vi "Builder.Main Thread.vi"(8 "error in (no error)":errorcluster, 10 "Thread Parameters":refnum<class "Thread Parameters.lvclass">, 11 "Builder in":refnum<class "Builder.lvclass">) -> (0 "error out":errorcluster, 3 "Builder out":refnum<class "Builder.lvclass">)   [LabVIEW 2016, in "DSF.Engine.lvlib" / "Builder.lvclass"]
uses:
  Builder.lvclass
  Thread Parameters/Thread Parameters.lvclass
  Thread Parameters/Thread Parameters.lvclass/Thread Parameters.ctl
  <vilib>/Platform/TimedLoop/XDataNode/timing_clust.ctl
  <vilib>/Platform/TimedLoop/XDataNode/nitl_modes.ctl
  <vilib>/Platform/TimedLoop/XDataNode/wakeup.ctl
  Builder.lvclass/Builder.ctl
  Interface/DSF.Engine.Interface.lvclass/DSF.Engine.Interface.ctl
  Interface/DSF.Engine.Interface.Builder.Response Data.ctl
  Interface/DSF.Engine.Interface.Builder.Response.ctl
  Interface/DSF.Engine.Interface.Builder.Read.Command.vi
  Interface/DSF.Engine.Interface.Builder.Write.Response.vi
  Interface/DSF.Engine.Interface.Get Command FIFO.vi
  Interface/DSF.Engine.Interface.RT FIFO.Read.vi
  Interface/DSF.Engine.Interface.RT FIFO.Write.vi
  Interface/DSF.Engine.Interface.Builder.lvclass
  C:/Git/Sourcetree/DSF/Source/Engine/Classes/Interface/DSF.Engine.Interface.lvclass
  <vilib>/platform/TimedLoop/XDataNode/XDataNode.xnode
  <vilib>/Platform/TimedLoop/XDataNode/XDNodeRunTimeDep.lvlib
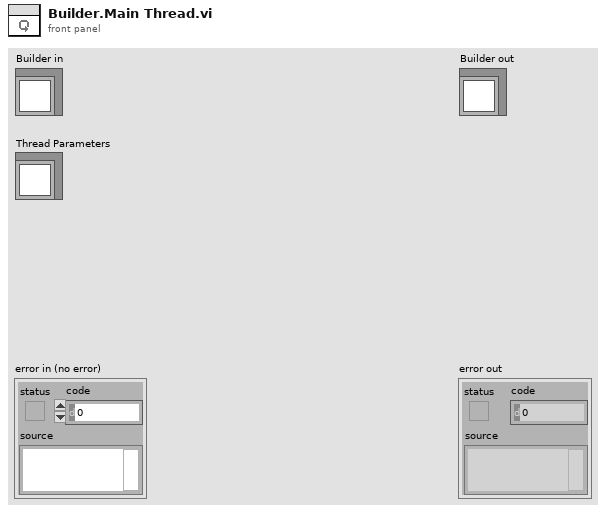
[diagram p1: front panel]
types:
  T1 = typedef "XDNodeRunTimeDep.lvlib/timing_clust.ctl" = cluster{"Expected End [f-1]":u64, "Actual End [f-1]":u64, "Finished Late? [f-1]":bool, "Expected End [i-1]":u64, "Actual End [i-1]":u64, "Finished Late? [i-1]":bool, "Expected Start [i]":u64, "Actual Start [i]":u64, "Expected Start [f]":u64, "Actual Start [f]":u64, "Source Name":string, "Structure Name":string, "Period":i64, "Deadline":i64, "Offset":i64, "Start":i64, "Priority":i32, "Timeout":i32, "Mode":T2, "Wakeup Reason":T3, "Error":errorcluster, "Source Type":string, "Secondary Source Type":string, "Global End Time":u64, "Global Start Time":u64, "Frame Duration":u64, "Iteration Duration":u64, "Assigned CPU":i32, "I/O Scan Engine Mode":u32}
  T2 = typedef "XDNodeRunTimeDep.lvlib/nitl_modes.ctl" = enum32{"No Change", "Process missed periods, maintain original phase", "Discard missed periods, maintain original phase", "Process missed periods, ignore original phase", "Discard missed periods, ignore original phase"}
  T3 = typedef "XDNodeRunTimeDep.lvlib/wakeup.ctl" = enum32{"Normal", "Aborted", "Asynchronous wakeup", "Timing source error", "Timed loop error", "Timeout"}
  T4 = typedef "DSF.Engine.lvlib/DSF.Engine.Interface.Builder.lvclass/DSF.Engine.Interface.Builder.Response Data.ctl" = cluster{"Response":T5, "Payload":u64}
  T5 = typedef "DSF.Engine.lvlib/DSF.Engine.Interface.Builder.lvclass/DSF.Engine.Interface.Builder.Response.ctl" = enum8{"General Ack", "Shutdown Ack"}
  T6 = typedef "DSF.Engine.lvlib/DSF.Engine.Interface.Builder.lvclass/DSF.Engine.Interface.Builder.Command Data.ctl" = cluster{"Command":T7, "Payload":u64}
  T7 = typedef "DSF.Engine.lvlib/DSF.Engine.Interface.Builder.lvclass/DSF.Engine.Interface.Builder.Command.ctl" = enum8{"Idle", "Initialize", "Build Buffer", "Parse Buffer", "Shutdown"}
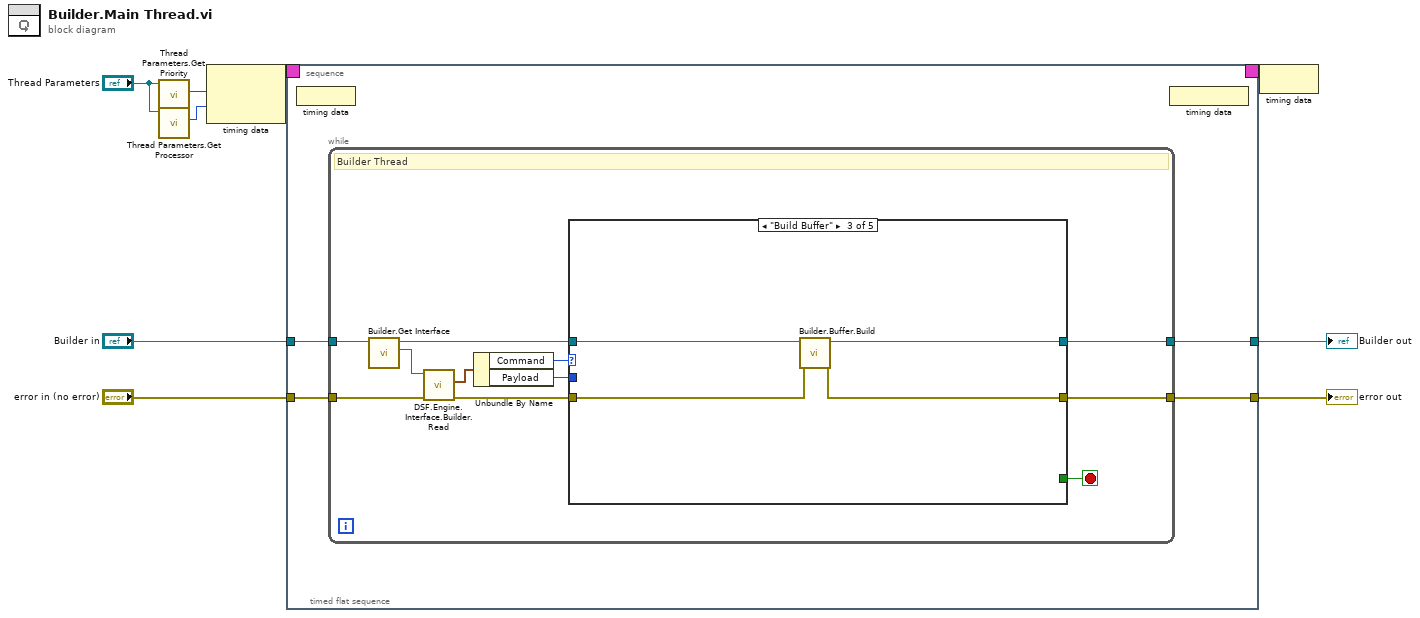
[diagram p0: block diagram]
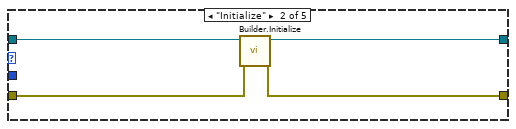
[diagram p3: hidden frame]
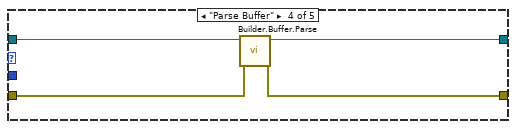
[diagram p4: hidden frame]
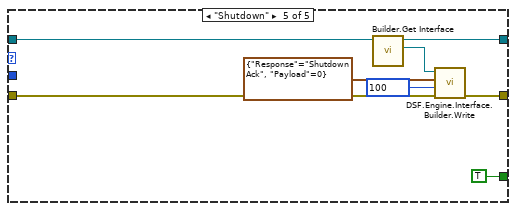
[diagram p5: hidden frame]
diagram:
  n1 = call "Thread Parameters.Get Priority.vi"("Thread Parameters in"="Thread Parameters") -> ("Priority"=w6:i32)  [unwired: 9 in, 1 out]
  n2 = call "Thread Parameters.Get Processor.vi"("Thread Parameters in"="Thread Parameters") -> ("Processor"=w5:i32)  [unwired: 9 in, 1 out]
  n3 = node-c288(w6, w5) -> (w8:T1)
  n4 = timed-sequence {
    timing: w8 -> [_]
    timing-out: [_] -> w7
    tunnel: "Builder in" -> [w12]
    tunnel: [w13] -> w4
    tunnel: "error in (no error)" -> [w11]
    tunnel: [w10] -> w2
    n5 = timed-flat-sequence {
      tunnel: [w17] -> w13
      tunnel: w12 -> [w15]
      tunnel: w11 -> [w16]
      tunnel: [w14] -> w10
      n6 = node-c288() -> ()  [unwired: 1 in]
      n7 = while {
        tunnel: w15 -> [w21]
        tunnel: [w25] -> w17
        tunnel: w16 -> [w29]
        tunnel: [w22] -> w14
        stop <- w20 stop-if-true
        # "Builder Thread"
        n8 = call "Builder.Get Interface.vi"("Builder in"=w21) -> ("Builder Interface"=w30:refnum<class "DSF.Engine.Interface.Builder.lvclass">, "Builder out"=w26:refnum<class "Builder.lvclass">)  [unwired: 9 in]
        n9 = call-poly "DSF.Engine.Interface.Builder.Read.vi"("error in (no error)"=w29, "Builder Interface in"=w30) -> ("error out"=w23:errorcluster, "command"=w28:T6)  [unwired: 5 in, 3 out]
        n10 = Unbundle By Name(w28) -> ("Command"=w27:T7, "Payload"=w24:u64)
        n11 = case shown="\"Build Buffer\"" w27 {
          tunnel: w26 -> [w32 w36 w40 w44 w52]
          tunnel: [w32 w35 w39 w43 w51] -> w25
          tunnel: w24 -> [_ _ _ _ _]
          tunnel: w23 -> [w31 w34 w38 w42 w47]
          tunnel: [w31 w33 w37 w41 w50] -> w22
          tunnel: [_ _ _ _ TRUE] -> w20
          frame "Idle", Default {
          }
          frame "Initialize" {
            n12 = call "Builder.Initialize.vi"("error in (no error)"=w34, "Builder in"=w36) -> ("error out"=w33:errorcluster, "Builder out"=w35:refnum<class "Builder.lvclass">)  [unwired: 8 in]
          }
          frame "Build Buffer" {
            n13 = call "Builder.Buffer.Build.vi"("error in (no error)"=w38, "Builder in"=w40) -> ("error out"=w37:errorcluster, "Builder out"=w39:refnum<class "Builder.lvclass">)  [unwired: 8 in]
          }
          frame "Parse Buffer" {
            n14 = call "Builder.Buffer.Parse.vi"("error in (no error)"=w42, "Builder in"=w44) -> ("error out"=w41:errorcluster, "Builder out"=w43:refnum<class "Builder.lvclass">)  [unwired: 8 in]
          }
          frame "Shutdown" {
            n15 = call "Builder.Get Interface.vi"("Builder in"=w52) -> ("Builder Interface"=w49:refnum<class "DSF.Engine.Interface.Builder.lvclass">, "Builder out"=w51:refnum<class "Builder.lvclass">)  [unwired: 9 in]
            n16 = call-poly "DSF.Engine.Interface.Builder.Write.vi"("error in (no error)"=w47, "timeout in ms (0)"=100, "response"=T4 {"Response"=enum."Shutdown Ack", "Payload"=0}, "Builder Interface in"=w49) -> ("error out"=w50:errorcluster)  [unwired: 5 in, 2 out]
          }
        }
      }
      n17 = node-c288() -> ()  [unwired: 1 out]
    }
  }
  "error out" <- w2
  "Builder out" <- w4
  n18 = node-c288(w7) -> ()
